vi "ExSubCloseCameraData.vi"(1 "error in (no error)":errorcluster, 2 "Image Handle":u32, 3 "Camera Handle":u32) -> (0 "error out":errorcluster)   [LabVIEW 2010]
panel:
  # "ExSubCloseCameraData:\nThis sub vi closes the camera handle and data handle."
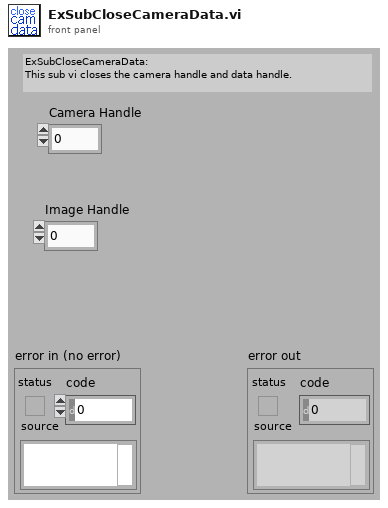
[diagram p1: front panel]
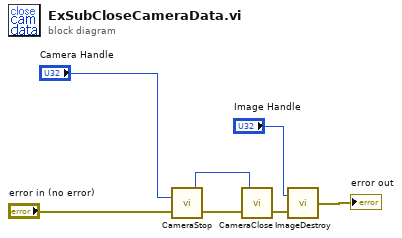
[diagram p0: block diagram]
diagram:
  n1 = call <userlib>:"CameraStop.vi"("error in"="error in (no error)", "Camera Handle"="Camera Handle") -> ("error out"=w3:errorcluster, "Camera Handle"=w7:u32)
  n2 = call <userlib>:"CameraClose.vi"("error in"=w3, "Camera Handle"=w7) -> ("error out"=w5:errorcluster)
  n3 = call <userlib>:"ImageDestroy.vi"("error in"=w5, "Data handle"="Image Handle") -> ("error out"=→"error out":errorcluster)
